vi "Wave2D_Cal Uk_Cal dt2 BC.vi"(10 "time step":i32, 11 "BC Value":dbl[][](array[numeric])) -> (3 "dt2 BC":dbl[](array[numeric]))   [LabVIEW 2020, in "NI_PDE.lvlib"]
uses:
  <vilib>/gmath/NI_PDE.lvlib
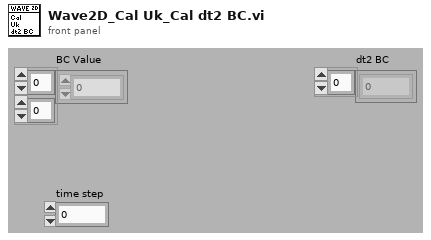
[diagram p1: front panel]
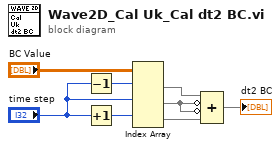
[diagram p0: block diagram]
diagram:
  n1 = Decrement(x="time step") -> (x-1=w7:i32)
  n2 = Increment(x="time step") -> (x+1=w6:i32)
  n3 = Index Array(array="BC Value", index (row) #1=w7, index (row) #2="time step", index (row) #3=w6) -> (element #1=w4:dbl[], element #2=w2:dbl[], element #3=w3:dbl[])  [unwired: 3 in]
  n4 = Compound Arithmetic op=ADD(w4, invert w2, invert w2, w3) -> (→"dt2 BC":dbl[])
